vi "CAN Unflatten.vi"(11 "Flatten Data in":u8[](array[numeric]) format="%.0x") -> (2 "Data":u8[](array[numeric]) format="%.0x", 3 "Header out":T1)   [LabVIEW 2021]
uses:
  typedef/FIFO Header.ctl
  <vilib>/CIF Foundation/CIF Utilities/DataTypes/Unflatten U64.vi
  <vilib>/CIF Foundation/CIF Utilities/DataTypes/Unflatten I64.vi
  ChannelCommon.lvlib
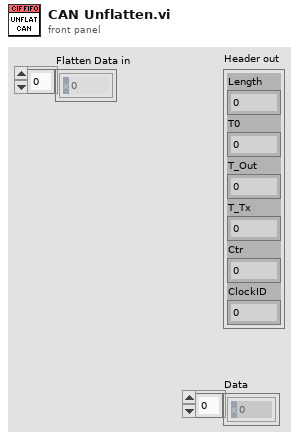
[diagram p1: front panel]
types:
  T1 = typedef "ChannelCommon.lvlib/FIFO Header.ctl" = cluster{"Length":u64, "T0":i64, "T_Out":i64, "T_Tx":i64, "Ctr":u64, "ClockID":u8}
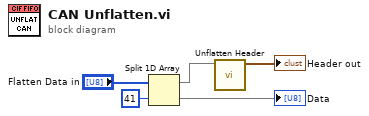
[diagram p0: block diagram]
diagram:
  n1 = Split 1D Array(array="Flatten Data in", index=41) -> (first subarray=w2:u8[], second subarray=→"Data":u8[])
  n2 = call "Unflatten Header.vi"("Flattened Data in"=w2) -> ("Header out"=→"Header out":T1)  [unwired: 9 in, 1 out]
